vi "Set Numeric With Type Preservation.vi"(10 "Numeric":i32, 11 "Parent in":refnum<class "Parent.lvclass">) -> (3 "Parent out":refnum<class "Parent.lvclass">)   [LabVIEW 2023, in "Parent.lvclass"]
doc: "In this VI, the Parent object does propagate from the input to the output terminal."
uses:
  Parent.lvclass
  Parent.lvclass/Parent.ctl
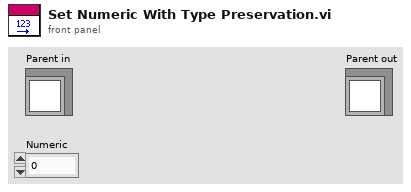
[diagram p1: front panel]
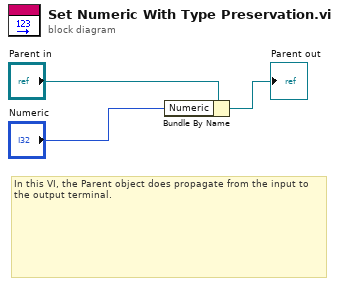
[diagram p0: block diagram]
diagram:
  # "In this VI, the Parent object does propagate from the input to the output terminal."
  n1 = Bundle By Name(cluster="Parent in", "Numeric"="Numeric") -> (→"Parent out":refnum<class "Parent.lvclass">)
